vi "validate configuration.vi"(8 "error in":errorcluster, 11 "TEC configuration in":refnum<class "TEC configuration.lvclass">) -> (0 "error out":errorcluster, 3 "TEC configuration out":refnum<class "TEC configuration.lvclass">)   [LabVIEW 2013, in "TEC configuration.lvclass"]
doc: "This function performs validation of the configuration. This function should be safe to call at any point and should not rely on anything in the runtime environment."
uses:
  TEC configuration.lvclass
  <vilib>/NI/Tag Bus Module Framework/module configuration/TBM module configuration.lvclass
  TEC configuration.lvclass/TEC configuration.ctl
  <vilib>/NI/Tag Bus Module Framework/root configuration/TBM configuration.lvclass
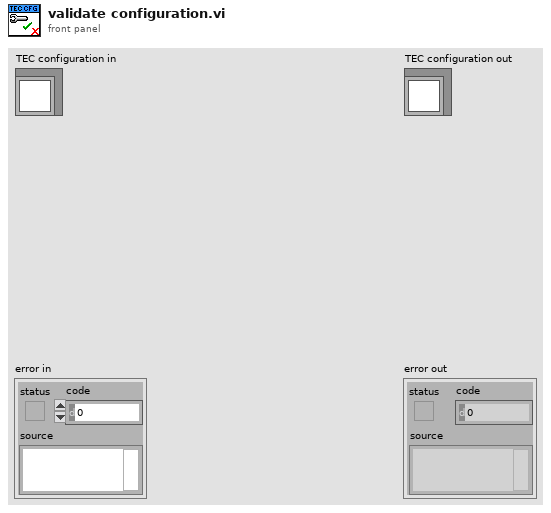
[diagram p1: front panel]
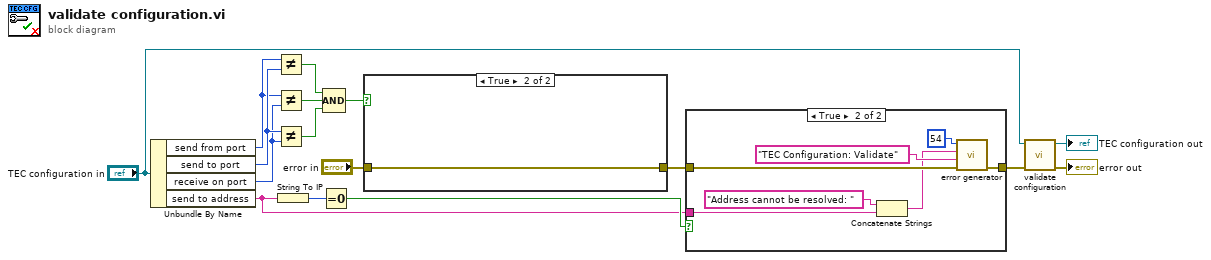
[diagram p0: block diagram]
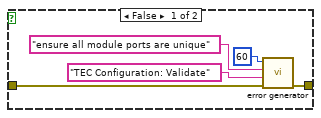
[diagram p3: hidden frame]
diagram:
  n1 = Unbundle By Name("TEC configuration in") -> ("send from port"=w12:u16, "send to port"=w13:u16, "receive on port"=w11:u16, "send to address"=w1:string)
  n2 = Not Equal?(x=w12, y=w13) -> (x != y?=w10:bool)
  n3 = Not Equal?(x=w12, y=w11) -> (x != y?=w9:bool)
  n4 = Not Equal?(x=w13, y=w11) -> (x != y?=w8:bool)
  n5 = String To IP(1:w1) -> (0:w3:u32)
  n6 = Equal To 0?(x=w3) -> (x = 0?=w2:bool)
  n7 = Compound Arithmetic op=AND(w10, w9, w8) -> (w7:bool)
  n8 = case shown="True" w7 {
    tunnel: [w20 w22] -> w5
    tunnel: "error in" -> [w21 w22]
    frame False {
      n9 = call <vilib>:"error generator.vi"("error in"=w21, "source"="TEC Configuration: Validate", "append error message"="ensure all module ports are unique", "error code (0)"=60) -> ("error out"=w20:errorcluster)  [unwired: 7 in]
    }
    frame True {
    }
  }
  n10 = case shown="True" w2 {
    tunnel: [w23 w29] -> w4
    tunnel: w5 -> [w23 w30]
    tunnel: w1 -> [_ w25]
    frame False {
    }
    frame True {
      n11 = Concatenate Strings("Address cannot be resolved: " ("string"), w25) -> (w24:string)
      n12 = call <vilib>:"error generator.vi"("error in"=w30, "source"="TEC Configuration: Validate", "append error message"=w24, "error code (0)"=54) -> ("error out"=w29:errorcluster)  [unwired: 7 in]
    }
  }
  n13 = call-parent "validate configuration.vi"("error in"=w4, "configuration in"="TEC configuration in") -> ("error out"=→"error out":errorcluster, "configuration out"=→"TEC configuration out":refnum<class "TEC configuration.lvclass">)  [unwired: 8 in]
